vi "Get Attribute Array as JSON.vi"(8 "error in":errorcluster, 10 "Attribute":string, 11 "Config from JSON in":refnum<class "Config from JSON.lvclass">) -> (0 "error out":errorcluster, 2 "<JSON>":string, 3 "Config from JSON out":refnum<class "Config from JSON.lvclass">)   [LabVIEW 2024, in "Config from JSON.lvclass"]
uses:
  Config from JSON.lvclass
  Config from JSON.lvclass/Config from JSON.ctl
  <vilib>/JDP Science/JSONtext/JSONtext.lvlib
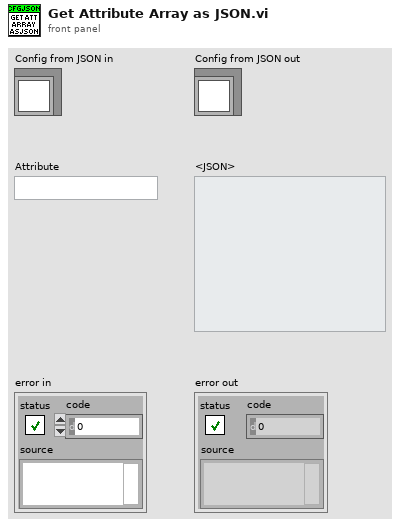
[diagram p1: front panel]
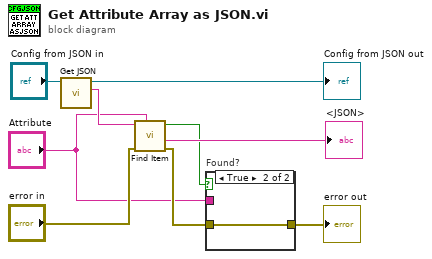
[diagram p0: block diagram]
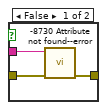
[diagram p2: hidden frame]
diagram:
  n1 = call-dynamic "Get JSON.vi"("ConfigFromJSON in"="Config from JSON in") -> ("<JSON>"=w7:string, "ConfigFromJSON out"=→"Config from JSON out":refnum<class "Config from JSON.lvclass">)  [unwired: 9 in]
  n2 = call <vilib>:"Find Item.vi"("$Path or Item Name"="Attribute", "error in (no error)"="error in", "JSON"=w7) -> ("error out"=w5:errorcluster, "<JSON>"=→"<JSON>":string, "Found"=w1:bool)  [unwired: 5 in, 1 out]
  n3 = case "Found?" shown="True" w1 {
    tunnel: w5 -> [w12 w13]
    tunnel: [w11 w13] -> w3
    tunnel: "Attribute" -> [w10 _]
    frame False {
      n4 = call "-8730 Attribute not found--error.vi"("error in"=w12, "Attribute"=w10) -> ("error out"=w11:errorcluster)  [unwired: 9 in]
    }
    frame True {
    }
  }
  "error out" <- w3
